vi "Read Timestamp.vi"(7 "field name":string="timeStamp", 8 "error in":errorcluster, 11 "Value in":refnum<class "Value.lvclass">) -> (0 "error out":errorcluster, 2 "timestamp":timestamp, 3 "Value out":refnum<class "Value.lvclass">)   [LabVIEW 2020, in "Value.lvlib" / "Value.lvclass"]
uses:
  Value.lvclass
  Value.lvclass/Value.ctl
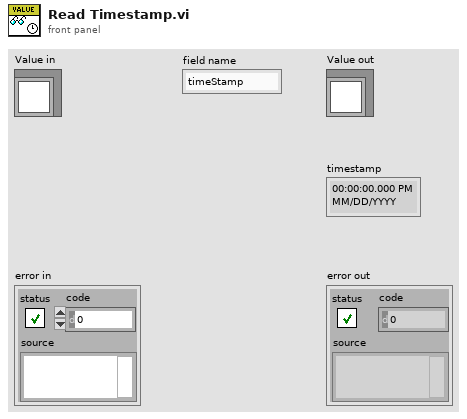
[diagram p1: front panel]
types:
  T1 = cluster{"seconds past epoch":i64, "nanoseconds":i32, "user tag":i32}
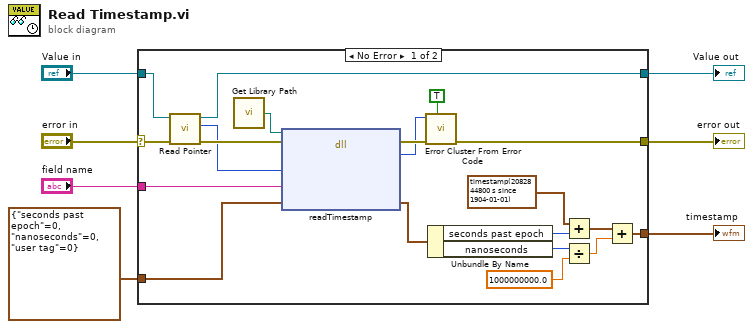
[diagram p0: block diagram]
diagram:
  n1 = case shown="No Error" "error in" {
    selector: "error in" -> [w22 w29]
    tunnel: [w23 w29] -> w7
    tunnel: "Value in" -> [w20 w28]
    tunnel: [w18 w28] -> w4
    tunnel: "field name" -> [w17 _]
    tunnel: T1 {"seconds past epoch"=0, "nanoseconds"=0, "user tag"=0} -> [w16 _]
    tunnel: [w8 _] -> w1
    frame No Error {
      n2 = call-dynamic "Read Pointer.vi"("error in (no error)"=w22, "Value in"=w20) -> ("error out"=w21:errorcluster, "pointer"=w19:i64, "Value out"=w18:refnum<class "Value.lvclass">)  [unwired: 7 in]
      n3 = call "Get Library Path.vi"() -> ("Path"=w27:path)  [unwired: 1 in]
      n4 = dll-call lib="?" fn="readTimestamp"(path in=w27, error in=w21, "value"=w19, "field_name"=w17, "timestamp"=w16) -> (error out=w25:errorcluster, "err_code"=w24:i32, "timestamp"=w15:T1)  [unwired: 3 in, 1 out]
      n5 = call <vilib>:"Error Cluster From Error Code.vi"("show call chain? (False)"=TRUE, "error in (no error)"=w25, "error code (0)"=w24) -> ("error out"=w23:errorcluster)  [unwired: 6 in]
      n6 = Unbundle By Name(w15) -> ("seconds past epoch"=w14:i64, "nanoseconds"=w11:i32)
      n7 = Add(x=timestamp(2082844800 s since 1904-01-01), y=w14) -> (x+y=w12:timestamp)
      n8 = Divide(x=w11, y=1000000000.0) -> (x/y=w9:dbl)
      n9 = Add(x=w12, y=w9) -> (x+y=w8:timestamp)
    }
    frame Error {
    }
  }
  "error out" <- w7
  "Value out" <- w4
  "timestamp" <- w1
